vi "Find DAQ Devices.vi"(8 "Error In":errorcluster) -> (0 "Error Out":errorcluster, 3 "DAQmx Device Name":tag)   [LabVIEW 2017]
doc: "This VI returns information on all DAQ devices connected to the development computer. \n\nIf you do not wire any of the search inputs it will not return an element. It will, however, return the list of connected devices and serial numbers and a table of all the devices connected."
uses:
  <resource>/objmgr/daqmx.rc
panel:
  in  "OK Button":bool=TRUE
  in  "ConnectedDevices":u16(ring) items=["Dev1", "Dev3"]
  out "All Device IDs":tag[](array[tag])
  # "Please select the correct connected device from the list:"
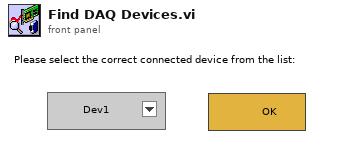
[diagram p1: front panel]
types:
  T1 = enum32{"Invalid", "Standard", "Closed", "Hidden", "Minimized", "Maximized"}
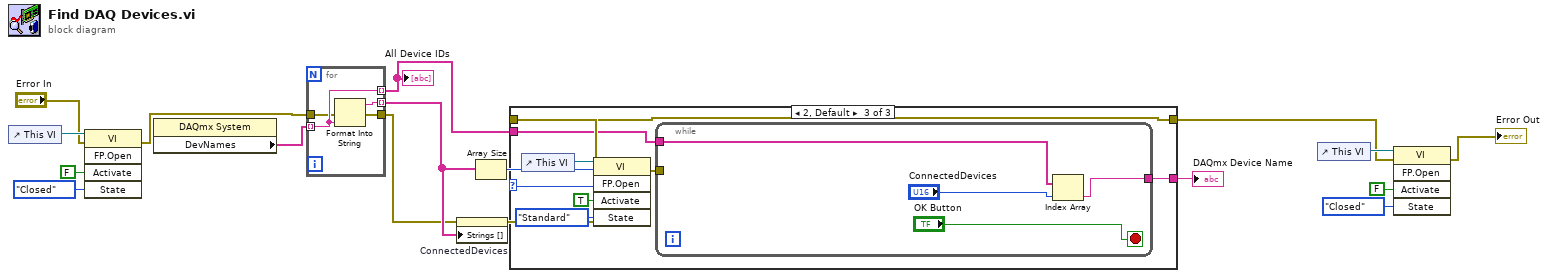
[diagram p0: block diagram]
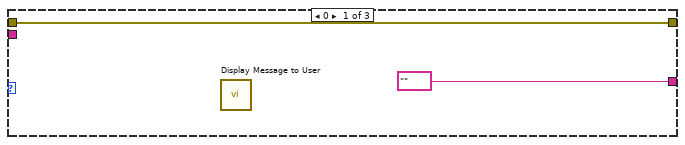
[diagram p2: hidden frame]
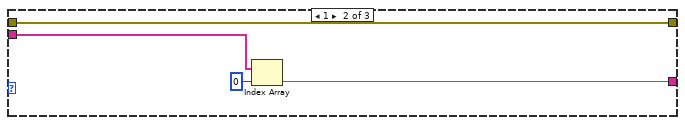
[diagram p3: hidden frame]
diagram:
  n1 = control-ref of="This VI"() -> (w5:refnum<vi>)
  n2 = invoke class="VI" method="FP.Open"(reference=w5, error in="Error In", "Activate"=FALSE ("Activate?"), "State"=T1."Closed") -> (error out=w3:errorcluster)  [unwired: 1 in, 4 out]
  n3 = property class="DAQmx System"() -> ("DevNames"=w17:tag[])  [unwired: 2 in, 2 out]
  n4 = for {
    tunnel: w17 -> [w20] mode=indexing
    tunnel: [w21] -> w16 mode=indexing
    tunnel: [w20] -> w14 mode=indexing
    tunnel: w3 -> [w19]
    tunnel: [w18] -> w2
    n5 = Format Into String(error in=w19, w20) -> (resulting string=w21:string, error out=w18:errorcluster)  [unwired: 2 in]
  }
  "All Device IDs" <- w14
  n6 = property on="ConnectedDevices" class="Ring (strict)"(error in=w2, "Strings []"=w16) -> (error out=w1:errorcluster)  [unwired: 1 in, 1 out]
  n7 = Array Size(array=w16) -> (size(s)=w15:i32)
  n8 = case shown="2, Default" w15 {
    tunnel: w14 -> [_ w27 w33]
    tunnel: [tag "" w25 w32] -> w13
    tunnel: w1 -> [w22 w24 w34]
    tunnel: [w22 w24 w34] -> w9
    frame 0 {
      n9 = call "Display Message to User"() -> ()  [unwired: 10 in, 2 out]
    }
    frame 1 {
      n10 = Index Array(array=w27, index=0) -> (element=w25:tag)
    }
    frame 2, Default {
      n11 = control-ref of="This VI"() -> (w29:refnum<vi>)
      n12 = invoke class="VI" method="FP.Open"(reference=w29, "Activate"=TRUE ("Activate?"), "State"=T1."Standard") -> (error out=w28:errorcluster)  [unwired: 2 in, 4 out]
      n13 = while {
        tunnel: w33 -> [w37]
        tunnel: [w36] -> w32
        tunnel: w28 -> [_]
        stop <- "OK Button" stop-if-true
        n14 = Index Array(array=w37, index="ConnectedDevices") -> (element=w36:tag)
      }
    }
  }
  "DAQmx Device Name" <- w13
  n15 = control-ref of="This VI"() -> (w10:refnum<vi>)
  n16 = invoke class="VI" method="FP.Open"(reference=w10, error in=w9, "Activate"=FALSE ("Activate?"), "State"=T1."Closed") -> (error out=→"Error Out":errorcluster)  [unwired: 1 in, 4 out]
